vi "sv_Check Data Valid [Octave Filtering].vi"(7 "reset filter (F)":bool, 8 "error in (no error)":errorcluster, 9 "midband frequency setting":T3, 10 "1/n octave settings":T2, 11 "scaled signal [EU]":waveform(dbl)) -> (0 "error out":errorcluster, 2 "reset filter":bool, 3 "dup scaled signal [EU]":waveform(dbl))   [LabVIEW 2017, in "SoundVib_Octave_2014 standard.lvlib"]
uses:
  <vilib>/addons/Sound and Vibration/svt_Octave/SoundVib_Octave_2014 standard.lvlib
  <vilib>/addons/_NISVFA/_Shared subVIs/Controls/svc_Octave Standard.ctl
  <vilib>/addons/_NISVFA/_Shared subVIs/Common/svc_Check for Waveform Parameter Continuity (no state).vi
  <vilib>/addons/_NISVFA/_Shared subVIs/Common/svc_Get SV Channel Info.vi
  <vilib>/addons/_NISVFA/_Shared subVIs/Common/svc_Engineering Units to Unit Label.vi
  <vilib>/addons/_NISVFA/_Shared subVIs/Common/svc_Unit Label to Engineering Units.vi
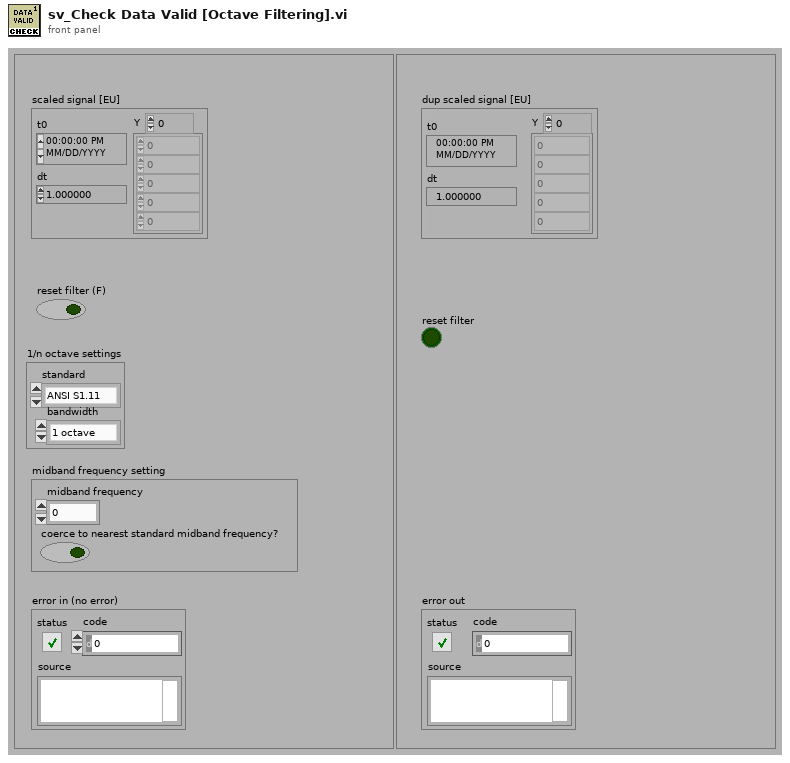
[diagram p1: front panel]
types:
  T1 = typedef "svc_Octave Standard.ctl" = enum16{"ANSI S1.11", "IEC 61260"}
  T2 = cluster{"standard":T1, "bandwidth":enum16{"1 octave", "1/3 octave", "1/6 octave", "1/12 octave", "1/24 octave"}}
  T3 = cluster{"midband frequency":dbl, "coerce to nearest standard midband frequency?":bool}
  T4 = cluster{"dt":bool, "t0 continuity":bool, "array length":bool, "channel info":bool, "name":bool}
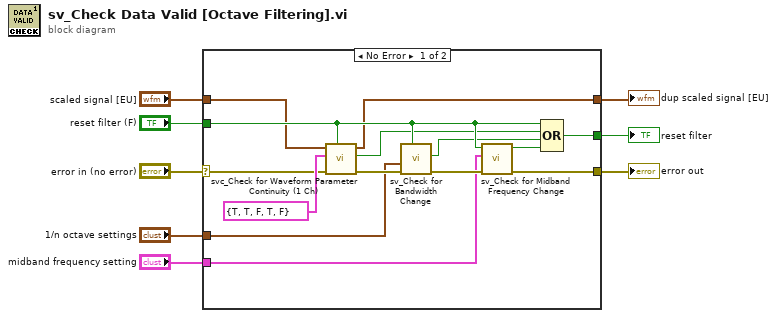
[diagram p0: block diagram]
diagram:
  n1 = case shown="No Error" "error in (no error)" {
    selector: "error in (no error)" -> [w18 w24]
    tunnel: "scaled signal [EU]" -> [w10 w23]
    tunnel: "reset filter (F)" -> [w16 w25]
    tunnel: "midband frequency setting" -> [w19 _]
    tunnel: "1/n octave settings" -> [w15 _]
    tunnel: [w12 w24] -> w3
    tunnel: [w11 w25] -> w2
    tunnel: [w9 w23] -> w1
    frame No Error {
      n2 = call <vilib>:"svc_Check for Waveform Parameter Continuity (1 Ch).vi"("restart averaging (F)"=w16, "error in (no error)"=w18, "checks for channel parameter change"=T4 {"dt"=TRUE, "t0 continuity"=TRUE, "array length"=FALSE, "channel info"=TRUE, "name"=FALSE}, "scaled signal [EU]"=w10) -> ("error out"=w21:errorcluster, "waveform parameter changed"=w14:bool, "dup scaled signal [EU]"=w9:waveform(dbl))  [unwired: 2 in, 3 out]
      n3 = call <vilib>:"sv_Check for Bandwidth Change.vi"("reset filter (F)"=w16, "error in (no error)"=w21, "1/n octave settings"=w15) -> ("error out"=w20:errorcluster, "parameter has changed"=w13:bool)  [unwired: 6 in, 1 out]
      n4 = call <vilib>:"sv_Check for Midband Frequency Change.vi"("error in (no error)"=w20, "midband frequency setting"=w19, "reset filter (F)"=w16) -> ("error out"=w12:errorcluster, "parameter has changed"=w17:bool)  [unwired: 7 in]
      n5 = Compound Arithmetic op=OR(w16, w14, w13, w17) -> (w11:bool)
    }
    frame Error {
    }
  }
  "error out" <- w3
  "reset filter" <- w2
  "dup scaled signal [EU]" <- w1
